vi "HoraUTC.vi"(0 "ENTRADA":string) -> (1 "hora utc":string, 2 "hora colombia":string)   [LabVIEW 2020]
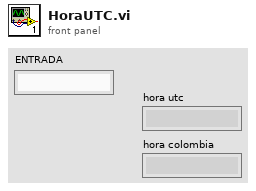
[diagram p1: front panel]
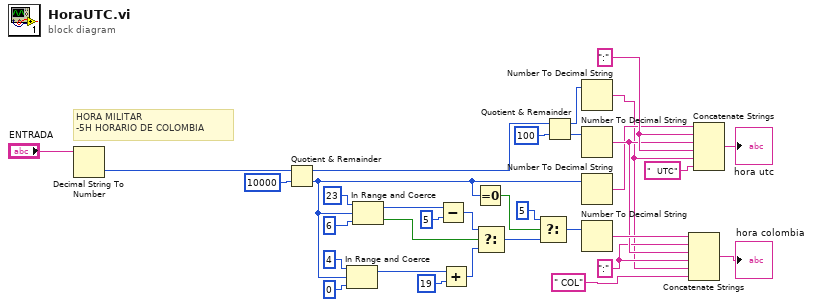
[diagram p0: block diagram]
diagram:
  w3 = ":"
  w10 = ":"
  # "HORA MILITAR \n-5H HORARIO DE COLOMBIA"
  n1 = Decimal String To Number(string="ENTRADA") -> (number=w25:i32)  [unwired: 2 in, 1 out]
  n2 = Quotient & Remainder(x=w25, y=10000) -> (x-y*floor(x/y)=w24:i32, floor(x/y)=w12:i32)
  n3 = In Range and Coerce(upper limit=4, x=w12, lower limit=0) -> (coerced(x)=w29:i32)  [unwired: 1 out]
  n4 = In Range and Coerce(upper limit=23, x=w12, lower limit=6) -> (coerced(x)=w27:i32, In Range?=w26:bool)
  n5 = Subtract(x=w27, y=5) -> (x-y=w28:i32)
  n6 = Add(x=w29, y=19) -> (x+y=w30:i32)
  n7 = Equal To 0?(x=w12) -> (x = 0?=w32:bool)
  n8 = Select(t=w28, s=w26, f=w30) -> (s? t:f=w31:i32)
  n9 = Select(t=5, s=w32, f=w31) -> (s? t:f=w11:i32)
  n10 = Quotient & Remainder(x=w24, y=100) -> (x-y*floor(x/y)=w14:i32, floor(x/y)=w13:i32)
  n11 = Number To Decimal String(number=w14) -> (decimal integer string=w2:string)  [unwired: 1 in]
  n12 = Number To Decimal String(number=w13) -> (decimal integer string=w5:string)  [unwired: 1 in]
  n13 = Number To Decimal String(number=w12) -> (decimal integer string=w4:string)  [unwired: 1 in]
  n14 = Number To Decimal String(number=w11) -> (decimal integer string=w6:string)  [unwired: 1 in]
  n15 = Concatenate Strings(w6, w3, w5, w3, w2, " COL" ("string")) -> (→"hora colombia":string)
  n16 = Concatenate Strings(w4, w10, w5, w10, w2, "  UTC" ("string")) -> (→"hora utc":string)
